vi "Release.vi"(8 "error in (no error)":errorcluster, 11 "SubscriptionDetails JSON in":refnum<class "SubscriptionDetails JSON.lvclass">) -> (0 "error out":errorcluster, 3 "SubscriptionDetails JSON out":refnum<class "SubscriptionDetails JSON.lvclass">)   [LabVIEW 2020, in "wamplv.lvlib" / "SubscriptionDetails JSON.lvclass"]
uses:
  SubscriptionDetails JSON.lvclass
  SubscriptionDetails JSON.lvclass/SubscriptionDetails JSON.ctl
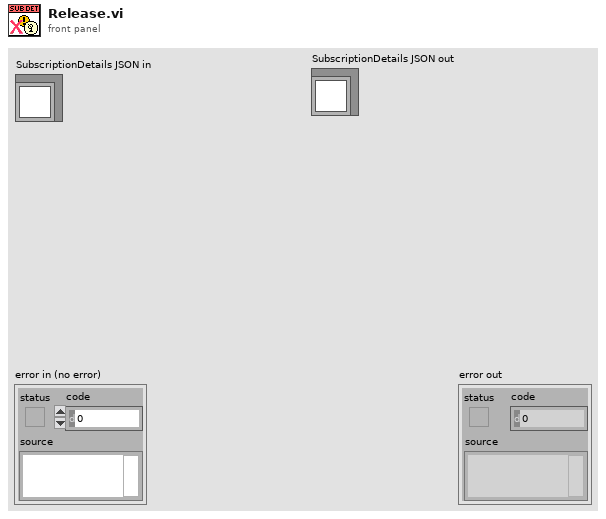
[diagram p1: front panel]
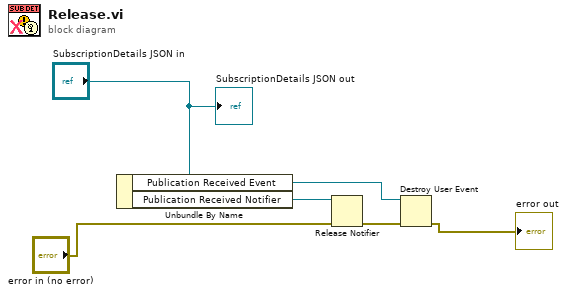
[diagram p0: block diagram]
diagram:
  n1 = Unbundle By Name("SubscriptionDetails JSON in") -> ("Publication Received Event"=w4:refnum<user-event>, "Publication Received Notifier"=w5:refnum<notifier>)
  n2 = Release Notifier(notifier=w5, error in (no error)="error in (no error)") -> (error out=w2:errorcluster)  [unwired: 1 in, 2 out]
  n3 = Destroy User Event(user event=w4, error in=w2) -> (error out=→"error out":errorcluster)
  "SubscriptionDetails JSON out" <- "SubscriptionDetails JSON in"
